vi "Set_4060_Watchdog_Timer.vi"(3 "Watchdog Timer  Seconds":i32 min=0 max=6553, 4 "Port Name":string="MainNetwork", 5 "Module Address":i32) -> (0 "Comment out":string, 1 "Reply":string, 2 "String to Write":string)   [LabVIEW 2010]
panel:
  # "Happy reply starts \"!\"\nUnhappy reply starts \"?\""
  # "\"0\" means Watchdog disabled"
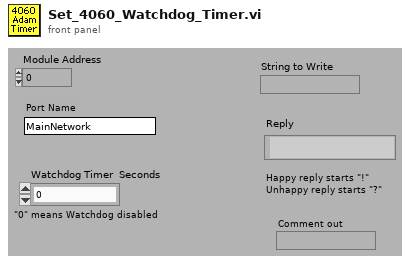
[diagram p1: front panel]
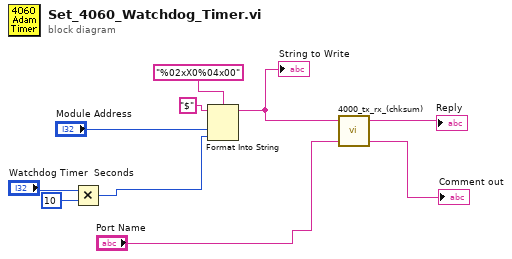
[diagram p0: block diagram]
diagram:
  n1 = Multiply(x="Watchdog Timer  Seconds", y=10) -> (x*y=w5:i32)
  n2 = Format Into String(format string="%02xX0%04x00", initial string="$", "Module Address", w5) -> (resulting string=w4:string)  [unwired: 1 in, 1 out]
  "String to Write" <- w4
  n3 = call "4000_tx_rx_(chksum).vi"("Port Name"="Port Name", "Write String"=w4) -> ("Comment out"=→"Comment out":string, "Read"=→"Reply":string)  [unwired: 1 in, 1 out]
